vi "Teleop.vi"(10 "Match Info":T7={"Autonomous Elapsed Seconds"=0.0, "TeleOp Elapsed Seconds"=0.0, "Disabled Elapsed Seconds"=0.0, "Visited Autonomous"=FALSE, "Visited TeleOp"=FALSE, "Visited Disabled"=FALSE, "Autonomous Settings"={"Autonomous Style"=enum."Independent", "VI Refnum"=refnum}}, 11 "Call Context":T8) -> ()   [LabVIEW 2013]
doc: "This VI is called for each TeleOp packet received from the DS where the robot is not disabled. It is often used to read from the joysticks and update I/O or to update setpoints for timed control loops. It should complete and return within 20 milliseconds or it may miss DS packets."
uses:
  <vilib>/Rock Robotics/WPI/DriverStation/WPI_DriverStationDerivedRobotMode.ctl
  <vilib>/Rock Robotics/WPI/DriverStation/WPI_DriverStationMatch Info.ctl
  <vilib>/Rock Robotics/WPI/Solenoid/WPI_SolenoidValue.ctl
  <vilib>/Rock Robotics/WPI/Relay/WPI_RelayValue.ctl
  Robot Global Data.vi
  <vilib>/Rock Robotics/Network Tables/SD Read Number.vi
  <vilib>/Rock Robotics/WPI/Joystick/WPI_JoystickGetSetRefNum.vi
  <vilib>/Rock Robotics/WPI/RobotDrive/WPI_RobotDriveGetSetRefNum.vi
  <vilib>/Rock Robotics/WPI/Solenoid/WPI_SolenoidSetEnum.vi
  <vilib>/Rock Robotics/WPI/Compressor/WPI_CompressorGetSetRefNum.vi
  <vilib>/Rock Robotics/WPI/Solenoid/WPI_SolenoidGetEnum.vi
panel:
  out "LockControls 2":bool
  in  "Mechanism Piston Forward 2":bool
  out "ManualOverridePistonStates":T2
  in  "TimingForCopilot":T3
  out "MovingBackwards":bool
  out "LockControls":bool
  out "MovingBackwardsEncoderReset":bool
  out "Waveform Chart 4":dbl(graph)
  out "Waveform Chart 3":dbl(graph)
  in  "Grabber Timer":dbl
  in  "GrabberCurrentTarget":dbl
  in  "HasGrabberBeenReset":bool
  in  "ToughBoxEncoderTopPosition":dbl
  in  "Current Grabber Status":T4(ring)
  in  "Run Grabber PID 2":bool
  out "Reed Switch 2":bool
  out "Reed Switch 1":bool
  out "Top Limit Tripped":bool
  out "Micro Switch":bool
  out "Bottom Limit Tripped":bool
  out "Axis Value  6":dbl
  out "Axis Value 5":dbl
  out "Axis Value 4":dbl
  in  "Grabber Axis Value":T5(ring)
  in  "Current Shooter Status":T6(ring)
  out "Waveform Chart":dbl(graph)
  out "Mechanism Moving Up":bool
  out "Mechanism Moving Down":bool
  out "Time Since Button Pressed":dbl
  in  "Manual Override Activated":bool
  in  "Button 2 Pressed":bool
  in  "Firing Pin Forward":bool
  in  "Mechanism Piston Forward":bool
  in  "Tick Taken":bool
  out "Time at Gather":dbl
  out "Timer for firing mech":dbl
  in  "Mechanism Status":string
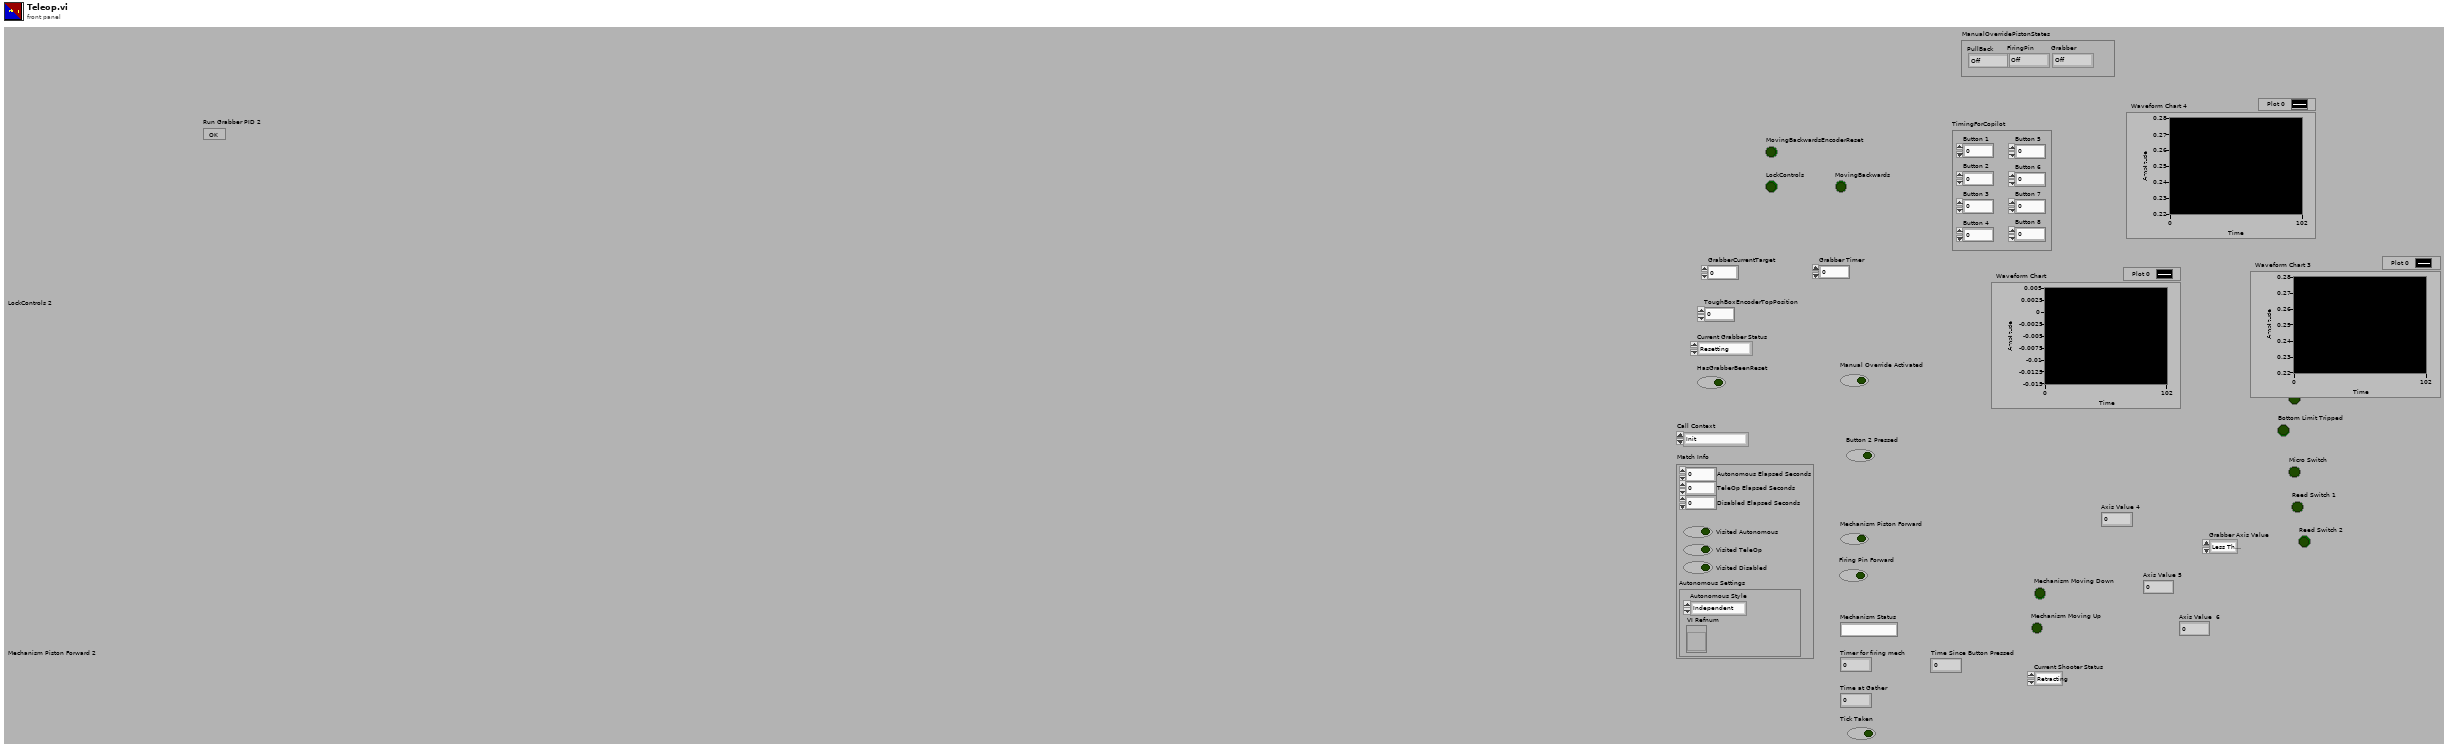
[diagram p1: front panel]
types:
  T1 = typedef "WPI_SolenoidValue.ctl" = enum16{"Off", "On", "Forward", "Reverse"}
  T2 = cluster{"PullBack":T1, "FiringPin":T1, "Grabber":T1}
  T3 = cluster{"Button 1":dbl, "Button 2":dbl, "Button 3":dbl, "Button 4":dbl, "Button 5":dbl, "Button 6":dbl, "Button 7":dbl, "Button 8":dbl}
  T4 = enum16{"Resetting", "Going Up", "Going Up Slow", "In Shooting Position", "Going Down", "Going Down Slow", "In Loading Position"}
  T5 = enum16{"Less Than Zero", "Greater Than Zero", "Equal To Zero"}
  T6 = enum16{"Retracting", "Firing", "Ready to fire", "Pulling back", "Just fired"}
  T7 = typedef "WPI_DriverStationMatch Info.ctl" = cluster{"Autonomous Elapsed Seconds":dbl, "TeleOp Elapsed Seconds":dbl, "Disabled Elapsed Seconds":dbl, "Visited Autonomous":bool, "Visited TeleOp":bool, "Visited Disabled":bool, "Autonomous Settings":cluster{"Autonomous Style":enum16{"Iterative", "Independent"}, "VI Refnum":refnum<vi>}}
  T8 = typedef "WPI_DriverStationDerivedRobotMode.ctl" = enum16{"Init", "Execute", "Stop"}
  T9 = enum16{"Resetting", "Going Up", "Going Up Slow", "In Shooting Position", "Going Down", "Going Down Slow", "In Loading Position", ""}
  T10 = typedef "WPI_JoystickDevRef.ctl" = cluster{"Device":T11}
  T11 = typedef "WPI_JoystickDeviceEnum.ctl" = enum16{"USB 1", "USB 2", "USB 3", "USB 4", "Kinect 1", "Kinect 2"}
  T12 = typedef "WPI_MotorControlDeviceRef.ctl" = cluster{"DeviceStatus":errorcluster, "Type":enum16{"PWM", "CAN"}, "PWM":cluster{"Digital Module":T13, "PWM Channel":T14, "DeadBand":T15}, "CAN":cluster{"Device Number":u8, "Control Mode":T16, "Semaphore":T17, "Max Vout":dbl}, "Invert":bool, "TransformRef":T18, "InvTransformRef":T18}
  T13 = typedef "FPGA_TypedefDigitalModule.ctl" = enum16{"Digital Module 1", "Digital Module 2"}
  T14 = typedef "FPGA_DIOPWMChannel.ctl" = enum8{"PWM 1", "PWM 2", "PWM 3", "PWM 4", "PWM 5", "PWM 6", "PWM 7", "PWM 8", "PWM 9", "PWM 10", "Invalid"}
  T15 = typedef "WPI_PWMDeadband.ctl" = cluster{"Name":string, "maxPositivePwm":i32, "minPositivePwm":i32, "centerPwm":i32, "maxNegativePwm":i32, "minNegativePwm":i32, "angularRange":u16}
  T16 = typedef "WPI_CANJaguar_ControlMode.ctl" = enum8{"Percent VBus", "Current", "Speed", "Position", "Voltage"}
  T17 = typedef "Semaphore RefNum" = refnum<k1>
  T18 = typedef "WPI_PWMTransform_ConPane.ctl" = refnum<vi>
  T19 = typedef "WPI_SolenoidDevRef.ctl" = cluster{"DevStatus":errorcluster, "Solenoid Module":T20, "Forward Solenoid Channel":T21, "Reverse Solenoid Channel":T21}
  T20 = typedef "FPGA_TypedefSolenoidModule.ctl" = enum16{"Solenoid Module 1", "Solenoid Module 2"}
  T21 = typedef "WPI_SolenoidChannel.ctl" = enum8{"Solenoid 1", "Solenoid 2", "Solenoid 3", "Solenoid 4", "Solenoid 5", "Solenoid 6", "Solenoid 7", "Solenoid 8", "Invalid"}
  T22 = typedef "WPI_JoystickButtonState.ctl" = cluster{"Button 1":bool, "Button 2":bool, "Button 3":bool, "Button 4":bool, "Button 5":bool, "Button 6":bool, "Button 7":bool, "Button 8":bool, "Button 9":bool, "Button 10":bool, "Button 11":bool, "Button 12":bool}
  T23 = typedef "WPI_DigitalInputDevRef.ctl" = cluster{"DevStatus":errorcluster, "DIO Channel":T24, "Digital Module":T13}
  T24 = typedef "FPGA_DIOChannel.ctl" = enum8{"DIO 1", "DIO 2", "DIO 3", "DIO 4", "DIO 5", "DIO 6", "DIO 7", "DIO 8", "DIO 9", "DIO 10", "DIO 11", "DIO 12", "DIO 13", "DIO 14", "Invalid"}
  T25 = typedef "WPI_EncoderDevRef.ctl" = cluster{"DevStatus":errorcluster, "EncoderIndex":T26, "CounterIndex":T27, "DistancePerCount":dbl, "Decoding Type":T28}
  T26 = typedef "FPGA_EncoderIdx.ctl" = enum8{"Enc 0", "Enc 1", "Enc 2", "Enc 3", "Invalid"}
  T27 = typedef "FPGA_CounterCtrSystemIndex.ctl" = enum8{"Ctr 0", "Ctr 1", "Ctr 2", "Ctr 3", "Ctr 4", "Ctr 5", "Ctr 6", "Ctr 7", "Invalid"}
  T28 = typedef "WPI_EncoderType.ctl" = enum16{"1x", "2x", "4x"}
  T29 = typedef "WPI_RelayDevRef.ctl" = cluster{"DevStatus":errorcluster, "Relay Channel":T30, "Digital Module":T13, "Relay Direction":T31}
  T30 = typedef "FPGA_DIORelayChannel.ctl" = enum8{"Relay 1", "Relay 2", "Relay 3", "Relay 4", "Relay 5", "Relay 6", "Relay 7", "Relay 8", "Invalid"}
  T31 = typedef "WPI_RelayDirection.ctl" = enum16{"Both directions", "Forward only", "Reverse only"}
  T32 = typedef "WPI_CompressorDevRef.ctl" = cluster{"DevStatus":errorcluster, "DigitalInputDevRef":T23, "RelayDevRef":T29}
  T33 = typedef "WPI_RelayValue.ctl" = enum16{"Off", "On", "Forward", "Reverse"}
  T34 = typedef "WPI_AnalogChannelDevRef.ctl" = cluster{"DevStatus":errorcluster, "Analog Module":T35, "Analog Channel":T36}
  T35 = typedef "FPGA_TypedefAnalogModule.ctl" = enum16{"Analog Module 1", "Analog Module 2"}
  T36 = typedef "FPGA_AIChannel.ctl" = enum8{"AI 1", "AI 2", "AI 3", "AI 4", "AI 5", "AI 6", "AI 7", "AI 8", "Invalid"}
  T37 = typedef "WPI_ServoDeviceRef.ctl" = cluster{"DeviceStatus":errorcluster, "Digital Module":T13, "PWM Channel":T14, "DeadBand":T15}
  T38 = cluster{"axis 1 (x)":dbl, "axis 2 (y)":dbl, "axis 3 (throttle)":dbl, "axis 4":dbl, "axis 5":dbl, "axis 6":dbl}
  T39 = typedef "WPI_RobotDriveDevRef.ctl" = cluster{"DevStatus":errorcluster, "Motors[]":T12[], "Square Inputs":bool, "Max Output":dbl, "Isochronous":bool}
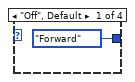
[diagram p3: hidden frame]
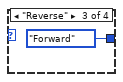
[diagram p4: hidden frame]
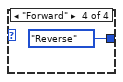
[diagram p5: hidden frame]
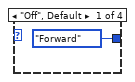
[diagram p7: hidden frame]
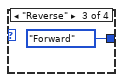
[diagram p8: hidden frame]
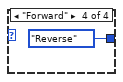
[diagram p9: hidden frame]
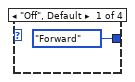
[diagram p11: hidden frame]
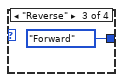
[diagram p12: hidden frame]
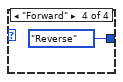
[diagram p13: hidden frame]
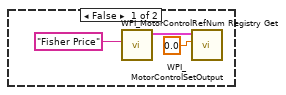
[diagram p15: hidden frame]
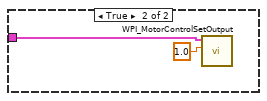
[diagram p16: hidden frame]
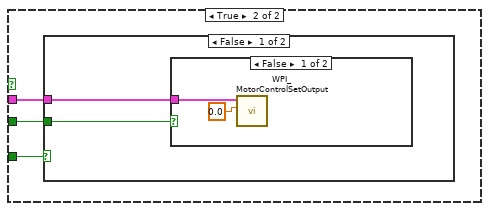
[diagram p17: hidden frame]
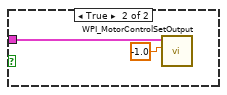
[diagram p18: hidden frame]
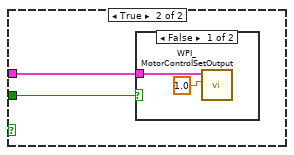
[diagram p19: hidden frame]
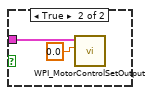
[diagram p20: hidden frame]
diagram:
  (unwired) FALSE
  (unwired) "This code sets the toggle rate used by the Periodic Tasks VI.  For teleop mode we flash the USER1 LED on the cRIO at a fast rate.  Look at the Periodic Tasks VI to see how this global value is used."
  (unwired) "This VI is called each time a TeleOp DS packet is received.  Use it to respond to new joystick or Driver Station values.\n\nCommon tasks include reading the joysticks and updating motors, and updating setpoints for periodic loops.\n\nYou can open I/O on the FIRST Call, or in the Begin.vi."
  # "Second joystick/copilot controls"
  # "Send information about the current state in the code to the drivers"
  # "one encoder"
  # "Top Limit Switch may need invert"
  # "one encoder"
  # "Check me!"
  # "Publish the Robot Drive Motor\nvalues to the dashboard"
  # "Each time we enter, report that\nwe are running teleop"
  # "Use to differentiate between\nFirst, Last, and Intermediate calls"
  # "Read Joystick X and Y values and update motor values"
  n1 = call <vilib>:"SD Read Boolean.vi"("Name"="Manual Mechanism Override") -> ("Boolean"=w100:bool)  [unwired: 8 in, 2 out]
  n2 = Not(x=w100) -> (.not. x?=w86:bool)
  n3 = local write "Firing Pin Forward"(FALSE) -> ()
  n4 = call <vilib>:"WPI_DriverStationReport Robot Code State.vi"("TeleOp"=TRUE ("Autonomous")) -> ()  [unwired: 10 in, 1 out]
  n5 = global write "Robot Global Data.vi" "LED toggle rate (ms)"(u32 100 ("LED ms toggle rate")) -> ()
  n6 = case shown="True" w86 {
    frame False {
    }
    frame True {
      n7 = local read "Current Grabber Status"() -> (w177:T4)
      n8 = case shown="\"Going Up Slow\"" w177 {
        frame "Going Up" {
          n9 = Divide(x=60.0 ("setpoint"), y=360.0) -> (x/y=w180:dbl)
          n10 = call "grabberpidinit.vi"("setpoint"=w180) -> ("Done? 2"=w181:bool)  [unwired: 10 in]
          n11 = case shown="True" w181 {
            tunnel: w180 -> [_ w182]
            frame False {
            }
            frame True {
              n12 = local write "GrabberCurrentTarget"(w182) -> ()
              n13 = local write "Current Grabber Status"(T4."Going Up Slow" ("Current Grabber Status")) -> ()
            }
          }
        }
        frame "In Loading Position" {
          # "Change to the UltraSonic Sensor\nwhen possible"
          n14 = call <vilib>:"WPI_JoystickRefNum Registry Get.vi"("refnum name"="Joystick 1") -> ("JoystickDevRef"=w186:T10)  [unwired: 1 in, 9 out]
          n15 = call <vilib>:"WPI_MotorControlRefNum Registry Get.vi"("refnum name"="Snowblower") -> ("MotorControlDevRef"=w193:T12)  [unwired: 9 in, 1 out]
          n16 = call <vilib>:"WPI_MotorControlSetOutput.vi"("Output"=1.0, "MotorControlDevRef"=w193) -> ()  [unwired: 7 in, 3 out]
          n17 = call <vilib>:"WPI_SolenoidRefNum Registry Get.vi"("refnum name"="Grabber Pistons Solenoid") -> ("error out"=w190:errorcluster, "SolenoidDevRef"=w189:T19)  [unwired: 9 in]
          n18 = call-poly <vilib>:"WPI_SolenoidSet.vi"("error in (no error)"=w190, "Value"=WPI_SolenoidValue."Reverse", "SolenoidDevRef"=w189) -> ()  [unwired: 7 in, 2 out]
          n19 = call <vilib>:"WPI_JoystickGet.vi"("JoystickDevRef"=w186) -> ("Buttons"=w185:T22)  [unwired: 1 in, 5 out]
          n20 = Unbundle By Name(w185) -> ("Button 4"=w184:bool)
          n21 = case shown="True" w184 {
            frame False {
            }
            frame True {
              n22 = local write "Current Grabber Status"(T4."Going Up" ("Current Grabber Status")) -> ()
            }
          }
        }
        frame "Going Down" {
          n23 = Divide(x=15.0, y=360.0) -> (x/y=w200:dbl)
          n24 = call "grabberpidinit.vi"("setpoint"=w200) -> ("Done? 2"=w201:bool)  [unwired: 10 in]
          n25 = case shown="True" w201 {
            tunnel: w200 -> [_ w206]
            frame False {
            }
            frame True {
              n26 = local write "GrabberCurrentTarget"(w206) -> ()
              n27 = local write "Current Grabber Status"(T4."Going Down Slow" ("Current Grabber Status")) -> ()
            }
          }
          n28 = call <vilib>:"WPI_DigitalInputRefNum Registry Get.vi"("refnum name"="Bottom Limit Switch") -> ("error out"=w198:errorcluster, "DigitalInputDevRef"=w197:T23)  [unwired: 9 in]
          n29 = call <vilib>:"WPI_DigitalInputGetValue.vi"("error in (no error)"=w198, "DigitalInputDevRef"=w197) -> ("Value"=w196:bool)  [unwired: 7 in, 2 out]
          n30 = case shown="True" w196 {
            frame False {
            }
            frame True {
              n31 = local write "Current Grabber Status"(T4."Going Down Slow" ("Current Grabber Status")) -> ()
            }
          }
        }
        frame "In Shooting Position" {
          n32 = call <vilib>:"WPI_JoystickRefNum Registry Get.vi"("refnum name"="Joystick 1") -> ("JoystickDevRef"=w209:T10)  [unwired: 1 in, 9 out]
          n33 = call <vilib>:"WPI_JoystickGet.vi"("JoystickDevRef"=w209) -> ("Buttons"=w208:T22)  [unwired: 1 in, 5 out]
          n34 = Unbundle By Name(w208) -> ("Button 1"=w207:bool)
          n35 = case shown="True" w207 {
            frame False {
            }
            frame True {
              n36 = local write "Current Grabber Status"(T9."Going Down" ("Current Grabber Status")) -> ()
            }
          }
        }
        frame "Going Down Slow" {
          n37 = call "grabberpidspeed.vi"("setpoint"=-20.0) -> ()  [unwired: 10 in, 1 out]
          n38 = call <vilib>:"WPI_DigitalInputRefNum Registry Get.vi"("refnum name"="Bottom Limit Switch") -> ("DigitalInputDevRef"=w214:T23)  [unwired: 9 in, 1 out]
          n39 = call <vilib>:"WPI_DigitalInputGetValue.vi"("DigitalInputDevRef"=w214) -> ("Value"=w213:bool)  [unwired: 8 in, 2 out]
          n40 = case shown="True" w213 {
            frame False {
            }
            frame True {
              n41 = local write "Current Grabber Status"(T4."In Loading Position" ("Current Grabber Status")) -> ()
            }
          }
        }
        frame "Going Up Slow" {
          n42 = call "grabberpidspeed.vi"("setpoint"=20.0) -> ()  [unwired: 10 in, 1 out]
          n43 = call <vilib>:"WPI_DigitalInputRefNum Registry Get.vi"("refnum name"="Top Limit Switch") -> ("DigitalInputDevRef"=w219:T23)  [unwired: 9 in, 1 out]
          n44 = call <vilib>:"WPI_DigitalInputGetValue.vi"("DigitalInputDevRef"=w219) -> ("Value"=w218:bool)  [unwired: 8 in, 2 out]
          n45 = case shown="True" w218 {
            frame False {
            }
            frame True {
              n46 = local write "Current Grabber Status"(T4."In Shooting Position" ("Current Grabber Status")) -> ()
            }
          }
        }
        frame "Resetting", Default {
          n47 = call "grabberpidspeed.vi"("setpoint"=-20.0) -> ()  [unwired: 10 in, 1 out]
          n48 = call <vilib>:"WPI_DigitalInputRefNum Registry Get.vi"("refnum name"="Bottom Limit Switch") -> ("DigitalInputDevRef"=w226:T23)  [unwired: 9 in, 1 out]
          n49 = call <vilib>:"WPI_DigitalInputGetValue.vi"("DigitalInputDevRef"=w226) -> ("Value"=w224:bool)  [unwired: 8 in, 2 out]
          n50 = Not(x=w224) -> (.not. x?=w223:bool)
          n51 = case shown="True" w223 {
            frame False {
            }
            frame True {
              n52 = local write "Current Grabber Status"(T9."In Loading Position" ("Current Grabber Status")) -> ()
              n53 = call <vilib>:"WPI_EncoderRefNum Registry Get.vi"("refnum name"="Tough Box Encoder") -> ("error out"=w229:errorcluster, "EncoderDevRef"=w228:T25)  [unwired: 9 in]
              n54 = call <vilib>:"WPI_EncoderReset.vi"("error in (no error)"=w229, "EncoderDevRef"=w228) -> ()  [unwired: 8 in, 2 out]
            }
          }
          n55 = Tick Count (ms)() -> ()  [unwired: 1 out]
        }
      }
    }
  }
  n56 = Unbundle By Name("Match Info") -> ()  [unwired: 1 out]
  n57 = call <vilib>:"SD Read Boolean.vi"("Name"="Light Ring On") -> ("Boolean"=w106:bool)  [unwired: 8 in, 2 out]
  n58 = call <vilib>:"WPI_RelayRefNum Registry Get.vi"("refnum name"="Light Ring") -> ("RelayDevRef"=w105:T29)  [unwired: 9 in, 1 out]
  n59 = call <vilib>:"WPI_DigitalInputRefNum Registry Get.vi"("refnum name"="Reed Switch 1") -> ("DigitalInputDevRef"=w124:T23)  [unwired: 9 in, 1 out]
  n60 = call <vilib>:"WPI_DigitalInputRefNum Registry Get.vi"("refnum name"="Reed Switch 2") -> ("DigitalInputDevRef"=w117:T23)  [unwired: 9 in, 1 out]
  n61 = call <vilib>:"WPI_DigitalInputRefNum Registry Get.vi"("refnum name"="Reed Switch 2") -> ("DigitalInputDevRef"=w121:T23)  [unwired: 9 in, 1 out]
  n62 = call <vilib>:"WPI_DigitalInputRefNum Registry Get.vi"("refnum name"="Micro Switch 1") -> ("DigitalInputDevRef"=w134:T23)  [unwired: 9 in, 1 out]
  n63 = call <vilib>:"WPI_DigitalInputRefNum Registry Get.vi"("refnum name"="Micro Switch 1") -> ("DigitalInputDevRef"=w113:T23)  [unwired: 9 in, 1 out]
  n64 = call <vilib>:"WPI_DigitalInputRefNum Registry Get.vi"("refnum name"="Top Limit Switch") -> ("DigitalInputDevRef"=w127:T23)  [unwired: 9 in, 1 out]
  n65 = call <vilib>:"SD Read Boolean.vi"("Name"="Compressor On/Off") -> ("Boolean"=w136:bool)  [unwired: 8 in, 2 out]
  n66 = call <vilib>:"WPI_CompressorRefNum Registry Get.vi"("refnum name"="Compressor") -> ("CompressorDevRef"=w137:T32)  [unwired: 9 in, 1 out]
  n67 = call <vilib>:"WPI_DigitalInputRefNum Registry Get.vi"("refnum name"="Bottom Limit Switch") -> ("DigitalInputDevRef"=w142:T23)  [unwired: 9 in, 1 out]
  n68 = case shown="False" w106 {
    tunnel: w105 -> [w231 w234]
    frame False {
      n69 = call <vilib>:"WPI_RelaySet.vi"("RelayValue"=WPI_RelayValue."Off", "RelayDevRef"=w231) -> ()  [unwired: 8 in, 2 out]
    }
    frame True {
      n70 = call <vilib>:"WPI_RelaySet.vi"("RelayValue"=WPI_RelayValue."Forward", "RelayDevRef"=w234) -> ()  [unwired: 8 in, 2 out]
    }
  }
  n71 = call <vilib>:"WPI_DigitalInputGetValue.vi"("DigitalInputDevRef"=w124) -> ("Value"=→"Reed Switch 1":bool)  [unwired: 8 in, 2 out]
  n72 = call <vilib>:"WPI_DigitalInputGetValue.vi"("DigitalInputDevRef"=w117) -> ("Value"=w116:bool)  [unwired: 8 in, 2 out]
  n73 = call <vilib>:"WPI_DigitalInputGetValue.vi"("DigitalInputDevRef"=w121) -> ("Value"=→"Reed Switch 2":bool)  [unwired: 8 in, 2 out]
  n74 = call <vilib>:"WPI_DigitalInputGetValue.vi"("DigitalInputDevRef"=w134) -> ("Value"=→"Micro Switch":bool)  [unwired: 8 in, 2 out]
  n75 = call <vilib>:"WPI_DigitalInputGetValue.vi"("DigitalInputDevRef"=w113) -> ("Value"=w112:bool)  [unwired: 8 in, 2 out]
  n76 = call <vilib>:"WPI_DigitalInputGetValue.vi"("DigitalInputDevRef"=w127) -> ("Value"=→"Top Limit Tripped":bool)  [unwired: 8 in, 2 out]
  n77 = call <vilib>:"WPI_AnalogChannelRefNum Registry Get.vi"("refnum name"="Grabber Ultrasonic Sensor") -> ("AIDeviceRef"=w103:T34)  [unwired: 9 in, 1 out]
  n78 = case shown="False" w136 {
    tunnel: w137 -> [w235 w236]
    frame False {
      n79 = call <vilib>:"WPI_CompressorStop.vi"("CompressorDevRef"=w235) -> ()  [unwired: 9 in, 2 out]
    }
    frame True {
      n80 = call <vilib>:"WPI_CompressorStart.vi"("CompressorDevRef"=w236) -> ()  [unwired: 9 in, 2 out]
    }
  }
  n81 = call <vilib>:"WPI_DigitalInputGetValue.vi"("DigitalInputDevRef"=w142) -> ("Value"=→"Bottom Limit Tripped":bool)  [unwired: 8 in, 2 out]
  n82 = Not(x=w116) -> (.not. x?=w115:bool)
  n83 = call-poly <vilib>:"SD Read Value.vi"("Name"="Camera Pitch Control") -> ("Numeric"=w151:dbl)  [unwired: 8 in, 2 out]
  n84 = Not(x=w112) -> (.not. x?=w111:bool)
  n85 = call <vilib>:"WPI_ServoRefNum Registry Get.vi"("refnum name"="Camera Pitch Servo") -> ("ServoDeviceRef"=w152:T37)  [unwired: 9 in, 1 out]
  n86 = call-poly <vilib>:"SD Read Value.vi"("Name"="Camera Rotation Control") -> ("Numeric"=w155:dbl)  [unwired: 8 in, 2 out]
  n87 = call <vilib>:"WPI_AnalogChannelGetVoltage.vi"("AIDeviceRef"=w103) -> ("Voltage"=→"Waveform Chart":dbl)  [unwired: 8 in, 2 out]
  n88 = call <vilib>:"WPI_ServoRefNum Registry Get.vi"("refnum name"="Camera Rotation Servo") -> ("ServoDeviceRef"=w154:T37)  [unwired: 9 in, 1 out]
  n89 = call <vilib>:"SD Write Boolean.vi"("Boolean"=w115, "Name"="Are Drawback Pistons Extended") -> ()  [unwired: 8 in, 2 out]
  n90 = call <vilib>:"SD Write Boolean.vi"("Boolean"=w111, "Name"="Is The Firing Pin Piston Extended") -> ()  [unwired: 8 in, 2 out]
  n91 = call <vilib>:"SD Read Boolean.vi"("Name"="Manual Mechanism Override") -> ("Boolean"=w145:bool)  [unwired: 8 in, 2 out]
  n92 = call <vilib>:"WPI_JoystickRefNum Registry Get.vi"("refnum name"="Joystick 1") -> ("JoystickDevRef"=w164:T10)  [unwired: 1 in, 9 out]
  n93 = call <vilib>:"WPI_ServoSetAngle.vi"("Angle"=w151, "ServoDeviceRef"=w152) -> ()  [unwired: 8 in, 2 out]
  n94 = call <vilib>:"WPI_ServoSetAngle.vi"("Angle"=w155, "ServoDeviceRef"=w154) -> ()  [unwired: 8 in, 2 out]
  n95 = call <vilib>:"SD Read Boolean.vi"("Name"="Drawback Pistons Activated") -> ("Boolean"=w131:bool)  [unwired: 8 in, 2 out]
  n96 = Not(x=w145) -> (.not. x?=w130:bool)
  n97 = call <vilib>:"WPI_JoystickGet.vi"("JoystickDevRef"=w164) -> ("Buttons"=w163:T22, "Axes"=w161:T38)  [unwired: 1 in, 4 out]
  n98 = call <vilib>:"WPI_JoystickRefNum Registry Get.vi"("refnum name"="Joystick 1") -> ("JoystickDevRef"=w80:T10)  [unwired: 1 in, 9 out]
  n99 = Unbundle By Name(w163) -> ("Button 3"=w93:bool, "Button 5"=w109:bool, "Button 6"=w110:bool)  [unwired: 2 out]
  n100 = And(x=w130, y=w131) -> (x .and. y?=w129:bool)
  n101 = Unbundle By Name(w161) -> ("axis 4"=→"Axis Value 4":dbl, "axis 5"=→"Axis Value 5":dbl, "axis 6"=→"Axis Value  6":dbl)
  n102 = call <vilib>:"WPI_MotorControlRefNum Registry Get.vi"("refnum name"="Snowblower") -> ("MotorControlDevRef"=w91:T12)  [unwired: 9 in, 1 out]
  n103 = local read "MovingBackwards"() -> (w75:bool)
  n104 = call <vilib>:"WPI_JoystickGet.vi"("JoystickDevRef"=w80) -> ("Buttons"=w79:T22)  [unwired: 1 in, 5 out]
  n105 = call <vilib>:"SD Read Boolean.vi"("Name"="Manual Mechanism Override") -> ("Boolean"=w73:bool)  [unwired: 8 in, 2 out]
  n106 = Unbundle By Name(w79) -> ("Button 3"=w76:bool)
  n107 = case shown="False" w73 {
    tunnel: w110 -> [_ w245]
    tunnel: w109 -> [w237 w244]
    tunnel: w91 -> [w238 w243]
    frame False {
      n108 = case shown="False" w237 {
        tunnel: w238 -> [w239 w241]
        frame False {
          n109 = call <vilib>:"WPI_MotorControlSetOutput.vi"("Output"=-1.0, "MotorControlDevRef"=w239) -> ()  [unwired: 7 in, 3 out]
        }
        frame True {
          n110 = call <vilib>:"WPI_MotorControlSetOutput.vi"("Output"=1.0, "MotorControlDevRef"=w241) -> ()  [unwired: 7 in, 3 out]
        }
      }
    }
    frame True {
      n111 = case shown="False" w245 {
        tunnel: w244 -> [w247 w253]
        tunnel: w243 -> [w246 w252]
        frame False {
          n112 = case shown="False" w247 {
            tunnel: w246 -> [w249 w251]
            frame False {
              n113 = call <vilib>:"WPI_MotorControlSetOutput.vi"("Output"=0.0, "MotorControlDevRef"=w249) -> ()  [unwired: 7 in, 3 out]
            }
            frame True {
              n114 = call <vilib>:"WPI_MotorControlSetOutput.vi"("Output"=-1.0, "MotorControlDevRef"=w251) -> ()  [unwired: 7 in, 3 out]
            }
          }
        }
        frame True {
          n115 = case shown="False" w253 {
            tunnel: w252 -> [w255 w257]
            frame False {
              n116 = call <vilib>:"WPI_MotorControlSetOutput.vi"("Output"=1.0, "MotorControlDevRef"=w255) -> ()  [unwired: 7 in, 3 out]
            }
            frame True {
              n117 = call <vilib>:"WPI_MotorControlSetOutput.vi"("Output"=0.0, "MotorControlDevRef"=w257) -> ()  [unwired: 7 in, 3 out]
            }
          }
        }
      }
    }
  }
  n118 = case shown="True" w75 {
    frame False {
      n119 = local write "LockControls"(FALSE) -> ()
    }
    frame True {
      n120 = local read "MovingBackwardsEncoderReset"() -> (w287:bool)
      n121 = local write "LockControls"(TRUE) -> ()
      n122 = call <vilib>:"WPI_EncoderRefNum Registry Get.vi"("refnum name"="Left Drive Encoder") -> ("error out"=w272:errorcluster, "EncoderDevRef"=w263:T25)  [unwired: 9 in]
      n123 = call <vilib>:"WPI_EncoderGet.vi"("error in (no error)"=w272, "EncoderDevRef"=w263) -> ("Distance"=w264:dbl)  [unwired: 4 in, 5 out]
      n124 = call <vilib>:"WPI_EncoderRefNum Registry Get.vi"("refnum name"="Right Drive Encoder") -> ("error out"=w273:errorcluster, "EncoderDevRef"=w274:T25)  [unwired: 9 in]
      n125 = call <vilib>:"WPI_EncoderGet.vi"("error in (no error)"=w273, "EncoderDevRef"=w274) -> ("Distance"=w276:dbl)  [unwired: 4 in, 5 out]
      n126 = Add(x=w264, y=w276) -> (x+y=w277:dbl)
      n127 = case shown="False" w287 {
        frame False {
          n128 = call <vilib>:"WPI_EncoderRefNum Registry Get.vi"("refnum name"="Left Drive Encoder") -> ("error out"=w300:errorcluster, "EncoderDevRef"=w299:T25)  [unwired: 9 in]
          n129 = call <vilib>:"WPI_EncoderRefNum Registry Get.vi"("refnum name"="Right Drive Encoder") -> ("error out"=w303:errorcluster, "EncoderDevRef"=w302:T25)  [unwired: 9 in]
          n130 = local write "MovingBackwardsEncoderReset"(TRUE ("MovingBackwardsEncoderReset")) -> ()
          n131 = call <vilib>:"WPI_EncoderReset.vi"("error in (no error)"=w300, "EncoderDevRef"=w299) -> ()  [unwired: 8 in, 2 out]
          n132 = call <vilib>:"WPI_EncoderReset.vi"("error in (no error)"=w303, "EncoderDevRef"=w302) -> ()  [unwired: 8 in, 2 out]
        }
        frame True {
        }
      }
      n133 = Divide(x=w277, y=2.0) -> (x/y=w281:dbl)
      n134 = call "distancepidinit.vi"("Distance From Target"=-8.0) -> ("Done?"=w259:bool)  [unwired: 10 in]
      n135 = case shown="True" w259 {
        frame False {
        }
        frame True {
          n136 = local write "MovingBackwardsEncoderReset"(FALSE ("MovingBackwardsEncoderReset")) -> ()
          n137 = local write "MovingBackwards"(FALSE ("MovingBackwards")) -> ()
        }
      }
      n138 = Multiply(x=6.0, y=3.141592653589793) -> (x*y=w284:dbl)
      n139 = Divide(x=w281, y=360.0) -> (x/y=w283:dbl)
      n140 = Multiply(x=w283, y=w284) -> (x*y=w285:dbl)
      n141 = Divide(x=w285, y=12.0) -> (x/y=w271:dbl)
      n142 = Multiply(x=w271, y=0.48) -> (x*y=w265:dbl)
      n143 = Greater?(x=w265, y=-5.0) -> (0:w266:bool)
      n144 = Greater?(x=w265, y=-4.0) -> (0:w268:bool)
      n145 = case shown="True" w266 {
        frame False {
        }
        frame True {
          n146 = call <vilib>:"WPI_SolenoidRefNum Registry Get.vi"("refnum name"="Firing Pin") -> ("error out"=w290:errorcluster, "SolenoidDevRef"=w291:T19)  [unwired: 9 in]
          n147 = call-poly <vilib>:"WPI_SolenoidSet.vi"("error in (no error)"=w290, "Value"=WPI_SolenoidValue."Reverse", "SolenoidDevRef"=w291) -> ()  [unwired: 7 in, 2 out]
        }
      }
      n148 = case shown="True" w268 {
        frame False {
        }
        frame True {
          n149 = call <vilib>:"WPI_SolenoidRefNum Registry Get.vi"("refnum name"="Grabber Pistons") -> ("error out"=w294:errorcluster, "SolenoidDevRef"=w295:T19)  [unwired: 9 in]
          n150 = call-poly <vilib>:"WPI_SolenoidSet.vi"("error in (no error)"=w294, "Value"=WPI_SolenoidValue."Forward", "SolenoidDevRef"=w295) -> ()  [unwired: 7 in, 2 out]
        }
      }
    }
  }
  n151 = case shown="True" w76 {
    frame False {
    }
    frame True {
      n152 = local write "MovingBackwards"(TRUE ("MovingBackwards")) -> ()
    }
  }
  n153 = local read "Current Grabber Status"() -> (w96:T4)
  n154 = local read "Current Shooter Status"() -> (w97:T6)
  n155 = case shown="True" w129 {
    tunnel: w93 -> [_ w306]
    frame False {
    }
    frame True {
      n156 = case shown="\"Pulling back\"" "Current Shooter Status" {
        tunnel: w306 -> [_ w314 _ _ _]
        frame "Firing" {
          n157 = Tick Count (ms)() -> (millisecond timer value=w308:u32)
          n158 = local write "Current Shooter Status"(T6."Just fired" ("Current Shooter Status")) -> ()
          n159 = call <vilib>:"WPI_SolenoidRefNum Registry Get.vi"("refnum name"="Firing Pin Solenoid") -> ("error out"=w312:errorcluster, "SolenoidDevRef"=w311:T19)  [unwired: 9 in]
          n160 = call-poly <vilib>:"WPI_SolenoidSet.vi"("error in (no error)"=w312, "Value"=WPI_SolenoidValue."Reverse", "SolenoidDevRef"=w311) -> ()  [unwired: 7 in, 2 out]
          n161 = local write "Timer for firing mech"(w308) -> ()
        }
        frame "Ready to fire" {
          # "Button one is pressed, so fire"
          n162 = case shown="True" w314 {
            frame False {
            }
            frame True {
              n163 = local write "Current Shooter Status"(T6."Firing" ("Current Shooter Status")) -> ()
            }
          }
        }
        frame "Pulling back" {
          # "Need to invert reed switch 2"
          n164 = call <vilib>:"WPI_DigitalInputRefNum Registry Get.vi"("refnum name"="Reed Switch 2") -> ("error out"=w317:errorcluster, "DigitalInputDevRef"=w318:T23)  [unwired: 9 in]
          n165 = call <vilib>:"WPI_DigitalInputGetValue.vi"("error in (no error)"=w317, "DigitalInputDevRef"=w318) -> ("Value"=w316:bool)  [unwired: 7 in, 2 out]
          n166 = call <vilib>:"WPI_SolenoidRefNum Registry Get.vi"("refnum name"="Drawback Pistons") -> ("error out"=w322:errorcluster, "SolenoidDevRef"=w321:T19)  [unwired: 9 in]
          n167 = call <vilib>:"WPI_SolenoidRefNum Registry Get.vi"("refnum name"="Firing Pin Solenoid") -> ("error out"=w326:errorcluster, "SolenoidDevRef"=w325:T19)  [unwired: 9 in]
          n168 = call-poly <vilib>:"WPI_SolenoidSet.vi"("error in (no error)"=w322, "Value"=WPI_SolenoidValue."Forward", "SolenoidDevRef"=w321) -> ()  [unwired: 7 in, 2 out]
          n169 = case shown="True" w316 {
            frame False {
            }
            frame True {
              n170 = Tick Count (ms)() -> (millisecond timer value=w328:u32)
              n171 = local write "Timer for firing mech"(w328) -> ()
              n172 = local write "Current Shooter Status"(T6."Retracting" ("Current Shooter Status")) -> ()
            }
          }
          n173 = call-poly <vilib>:"WPI_SolenoidSet.vi"("error in (no error)"=w326, "Value"=WPI_SolenoidValue."Reverse", "SolenoidDevRef"=w325) -> ()  [unwired: 7 in, 2 out]
        }
        frame "Retracting" {
          n174 = local read "Timer for firing mech"() -> (w343:dbl)
          n175 = call <vilib>:"WPI_DigitalInputRefNum Registry Get.vi"("refnum name"="Reed Switch 1") -> ("error out"=w337:errorcluster, "DigitalInputDevRef"=w338:T23)  [unwired: 9 in]
          n176 = call <vilib>:"WPI_DigitalInputGetValue.vi"("error in (no error)"=w337, "DigitalInputDevRef"=w338) -> ("Value"=w330:bool)  [unwired: 7 in, 2 out]
          n177 = call <vilib>:"WPI_SolenoidRefNum Registry Get.vi"("refnum name"="Firing Pin Solenoid") -> ("error out"=w346:errorcluster, "SolenoidDevRef"=w345:T19)  [unwired: 9 in]
          n178 = Not(x=w330) -> (.not. x?=w331:bool)
          n179 = call-poly <vilib>:"WPI_SolenoidSet.vi"("error in (no error)"=w346, "Value"=WPI_SolenoidValue."Forward", "SolenoidDevRef"=w345) -> ()  [unwired: 7 in, 2 out]
          n180 = Tick Count (ms)() -> (millisecond timer value=w342:u32)
          n181 = case shown="True" w331 {
            frame False {
            }
            frame True {
              n182 = local write "Current Shooter Status"(T6."Ready to fire" ("Current Shooter Status")) -> ()
            }
          }
          n183 = Subtract(x=w342, y=w343) -> (x-y=w333:dbl)
          n184 = Greater Or Equal?(x=w333, y=1000) -> (x >= y?=w335:bool)
          n185 = call <vilib>:"WPI_SolenoidRefNum Registry Get.vi"("refnum name"="Drawback Pistons") -> ("SolenoidDevRef"=w340:T19)  [unwired: 9 in, 1 out]
          n186 = And(x=TRUE, y=w335) -> (x .and. y?=w336:bool)
          n187 = case shown="False" w336 {
            tunnel: w340 -> [w349 w351]
            frame False {
              n188 = call-poly <vilib>:"WPI_SolenoidSet.vi"("Value"=WPI_SolenoidValue."Forward", "SolenoidDevRef"=w349) -> ()  [unwired: 8 in, 2 out]
            }
            frame True {
              n189 = call-poly <vilib>:"WPI_SolenoidSet.vi"("Value"=WPI_SolenoidValue."Reverse", "SolenoidDevRef"=w351) -> ()  [unwired: 8 in, 2 out]
            }
          }
        }
        frame "Just fired", Default {
          # "When MicroSwitch is \nadded, Change this \nto read from that"
          n190 = local read "Timer for firing mech"() -> (w363:dbl)
          n191 = call <vilib>:"WPI_SolenoidRefNum Registry Get.vi"("refnum name"="Firing Pin Solenoid") -> ("error out"=w360:errorcluster, "SolenoidDevRef"=w359:T19)  [unwired: 9 in]
          n192 = Tick Count (ms)() -> (millisecond timer value=w362:u32)
          n193 = call-poly <vilib>:"WPI_SolenoidSet.vi"("error in (no error)"=w360, "Value"=WPI_SolenoidValue."Reverse", "SolenoidDevRef"=w359) -> ()  [unwired: 7 in, 2 out]
          n194 = Subtract(x=w362, y=w363) -> (x-y=w354:dbl)
          n195 = Greater Or Equal?(x=w354, y=3000) -> (x >= y?=w357:bool)
          n196 = And(x=TRUE, y=w357) -> (x .and. y?=w356:bool)
          n197 = case shown="True" w356 {
            frame False {
            }
            frame True {
              n198 = local write "Current Shooter Status"(T6."Pulling back" ("Current Shooter Status")) -> ()
            }
          }
        }
      }
    }
  }
  n199 = case shown="\"Resetting\", Default" w96 {
    tunnel: ["Resetting" "Going Up" "Going Up Slow" "In Shooting Position" "Going Down" "Going Down Slow" "In Loading Position"] -> w95
    frame "Resetting", Default {
    }
    frame "Going Up" {
    }
    frame "Going Up Slow" {
    }
    frame "In Shooting Position" {
    }
    frame "Going Down" {
    }
    frame "Going Down Slow" {
    }
    frame "In Loading Position" {
    }
  }
  n200 = case shown="\"Retracting\", Default" w97 {
    tunnel: ["Retracting" "Firing" "Ready to fire" "Pulling back" "Just fired"] -> w94
    frame "Retracting", Default {
    }
    frame "Firing" {
    }
    frame "Ready to fire" {
    }
    frame "Pulling back" {
    }
    frame "Just fired" {
    }
  }
  n201 = call <vilib>:"SD Write String.vi"("String"=w94, "Name"="Current Shooter Status") -> ()  [unwired: 8 in, 2 out]
  n202 = call <vilib>:"SD Write String.vi"("String"=w95, "Name"="Current Grabber Status") -> ()  [unwired: 8 in, 2 out]
  n203 = call <vilib>:"WPI_EncoderRefNum Registry Get.vi"("refnum name"="Right Drive Encoder") -> ("error out"=w90:errorcluster, "EncoderDevRef"=w89:T25)  [unwired: 9 in]
  n204 = call <vilib>:"WPI_EncoderGet.vi"("error in (no error)"=w90, "EncoderDevRef"=w89) -> ("Distance"=→"Waveform Chart 4":dbl)  [unwired: 4 in, 5 out]
  n205 = call <vilib>:"WPI_JoystickRefNum Registry Get.vi"("refnum name"="Joystick 2") -> ("JoystickDevRef"=w71:T10)  [unwired: 1 in, 9 out]
  n206 = call <vilib>:"WPI_JoystickGet.vi"("JoystickDevRef"=w71) -> ("Buttons"=w70:T22, "Axes"=w51:T38)  [unwired: 1 in, 4 out]
  n207 = Unbundle By Name(w51) -> ("axis 3 (throttle)"=w44:dbl, "axis 5"=w50:dbl)
  n208 = Negate(x=w50) -> (-x=w49:dbl)
  n209 = Multiply(x=w49, y=0.75) -> (x*y=w47:dbl)
  n210 = call <vilib>:"WPI_DigitalInputRefNum Registry Get.vi"("refnum name"="Micro Switch 1") -> ("DigitalInputDevRef"=w63:T23)  [unwired: 9 in, 1 out]
  n211 = Unbundle By Name(w70) -> ("Button 1"=w29:bool, "Button 2"=w11:bool, "Button 3"=w2:bool)  [unwired: 1 out]
  n212 = call <vilib>:"WPI_DigitalInputRefNum Registry Get.vi"("refnum name"="Bottom Limit Switch") -> ("DigitalInputDevRef"=w67:T23)  [unwired: 9 in, 1 out]
  n213 = call <vilib>:"WPI_DigitalInputGetValue.vi"("DigitalInputDevRef"=w63) -> ("Value"=w64:bool)  [unwired: 8 in, 2 out]
  n214 = call <vilib>:"WPI_DigitalInputRefNum Registry Get.vi"("refnum name"="Top Limit Switch") -> ("DigitalInputDevRef"=w60:T23)  [unwired: 9 in, 1 out]
  n215 = call <vilib>:"WPI_DigitalInputGetValue.vi"("DigitalInputDevRef"=w67) -> ("Value"=w55:bool)  [unwired: 8 in, 2 out]
  n216 = call <vilib>:"WPI_DigitalInputGetValue.vi"("DigitalInputDevRef"=w60) -> ("Value"=w52:bool)  [unwired: 8 in, 2 out]
  n217 = Not(x=w64) -> (.not. x?=w54:bool)
  n218 = Multiply(x=w44, y=0.4) -> (x*y=w45:dbl)
  n219 = local read "TimingForCopilot"() -> (w28:T3)
  n220 = Add(x=w47, y=w45) -> (x+y=w46:dbl)
  n221 = And(x=w55, y=w54) -> (x .and. y?=w53:bool)
  n222 = And(x=w52, y=w54) -> (x .and. y?=w58:bool)
  n223 = call <vilib>:"WPI_EncoderRefNum Registry Get.vi"("refnum name"="Tough Box Encoder") -> ("error out"=w85:errorcluster, "EncoderDevRef"=w84:T25)  [unwired: 9 in]
  n224 = Greater?(x=w46, y=0.01) -> (0:w59:bool)
  n225 = Less?(x=w46, y=-0.01) -> (x < y?=w66:bool)
  n226 = call <vilib>:"WPI_EncoderGet.vi"("error in (no error)"=w85, "EncoderDevRef"=w84) -> ("Distance"=→"Waveform Chart 3":dbl)  [unwired: 4 in, 5 out]
  n227 = And(x=w59, y=w58) -> (x .and. y?=w57:bool)
  n228 = Unbundle By Name(w28) -> ("Button 1"=w27:dbl, "Button 2"=w10:dbl, "Button 3"=w3:dbl)
  n229 = call <vilib>:"SD Read Boolean.vi"("Name"="Manual Mechanism Override") -> ("Boolean"=w36:bool)  [unwired: 8 in, 2 out]
  n230 = And(x=w53, y=w66) -> (x .and. y?=w56:bool)
  n231 = local read "LockControls"() -> (w78:bool)
  n232 = local read "ManualOverridePistonStates"() -> (w1:T2)
  n233 = Or(x=w56, y=w57) -> (x .or. y?=w41:bool)
  n234 = Tick Count (ms)() -> (millisecond timer value=w34:u32)
  n235 = Tick Count (ms)() -> (millisecond timer value=w21:u32)
  n236 = Tick Count (ms)() -> (millisecond timer value=w16:u32)
  n237 = call <vilib>:"SD Read Boolean.vi"("Name"="Grabber Limits Disabled") -> ("Boolean"=w39:bool)  [unwired: 8 in, 2 out]
  n238 = local read "Manual Override Activated"() -> (w37:bool)
  n239 = Or(x=w41, y=w39) -> (x .or. y?=w42:bool)
  n240 = Subtract(x=w34, y=w27) -> (x-y=w33:dbl)
  n241 = Subtract(x=w21, y=w10) -> (x-y=w20:dbl)
  n242 = Subtract(x=w16, y=w3) -> (x-y=w15:dbl)
  n243 = Not(x=w78) -> (.not. x?=w77:bool)
  n244 = Not Equal?(x=w37, y=w36) -> (x != y?=w35:bool)
  n245 = Greater?(x=w33, y=400.0) -> (0:w30:bool)
  n246 = Greater?(x=w20, y=400.0) -> (0:w17:bool)
  n247 = Greater?(x=w15, y=400.0) -> (0:w12:bool)
  n248 = Unbundle By Name(w1) -> ("PullBack"=w23:T1, "FiringPin"=w8:T1, "Grabber"=w4:T1)
  n249 = And(x=w30, y=w29) -> (x .and. y?=w31:bool)
  n250 = And(x=w17, y=w11) -> (x .and. y?=w18:bool)
  n251 = And(x=w12, y=w2) -> (x .and. y?=w13:bool)
  n252 = flat-sequence {
    tunnel: w35 -> [w377]
    frame #0 {
      n253 = case shown="True" w377 {
        frame False {
        }
        frame True {
          n254 = call <vilib>:"WPI_SolenoidRefNum Registry Get.vi"("refnum name"="Firing Pin") -> ("error out"=w384:errorcluster, "SolenoidDevRef"=w383:T19)  [unwired: 9 in]
          n255 = local read "ManualOverridePistonStates"() -> (w391:T2)
          n256 = call-poly <vilib>:"WPI_SolenoidGet.vi"("error in (no error)"=w384, "SolenoidDevRef"=w383) -> ("Value"=w382:T1)  [unwired: 7 in, 2 out]
          n257 = call <vilib>:"WPI_SolenoidRefNum Registry Get.vi"("refnum name"="Drawback Pistons") -> ("error out"=w388:errorcluster, "SolenoidDevRef"=w387:T19)  [unwired: 9 in]
          n258 = call <vilib>:"WPI_SolenoidRefNum Registry Get.vi"("refnum name"="Grabber Pistons") -> ("error out"=w380:errorcluster, "SolenoidDevRef"=w379:T19)  [unwired: 9 in]
          n259 = call-poly <vilib>:"WPI_SolenoidGet.vi"("error in (no error)"=w388, "SolenoidDevRef"=w387) -> ("Value"=w386:T1)  [unwired: 7 in, 2 out]
          n260 = call-poly <vilib>:"WPI_SolenoidGet.vi"("error in (no error)"=w380, "SolenoidDevRef"=w379) -> ("Value"=w378:T1)  [unwired: 7 in, 2 out]
          n261 = Bundle By Name(cluster=w391, "PullBack"=w386, "FiringPin"=w382, "Grabber"=w378) -> (w390:T2)
          n262 = local write "ManualOverridePistonStates"(w390) -> ()
        }
      }
    }
  }
  n263 = case shown="True" w31 {
    tunnel: w27 -> [w393 _]
    tunnel: [w393 w396] -> w26
    tunnel: w23 -> [w392 w395]
    tunnel: [w392 w394] -> w22
    frame False {
    }
    frame True {
      n264 = case shown="\"On\"" w395 {
        tunnel: [WPI_SolenoidValue."Forward" ("FiringPin") WPI_SolenoidValue."Reverse" ("FiringPin") WPI_SolenoidValue."Forward" ("FiringPin") WPI_SolenoidValue."Reverse" ("FiringPin")] -> w394
        frame "Off", Default {
        }
        frame "On" {
        }
        frame "Reverse" {
        }
        frame "Forward" {
        }
      }
      n265 = Tick Count (ms)() -> (millisecond timer value=w396:u32)
    }
  }
  n266 = case shown="True" w18 {
    tunnel: w10 -> [w402 _]
    tunnel: [w402 w405] -> w9
    tunnel: w8 -> [w401 w404]
    tunnel: [w401 w403] -> w7
    frame False {
    }
    frame True {
      n267 = case shown="\"On\"" w404 {
        tunnel: [WPI_SolenoidValue."Forward" ("FiringPin") WPI_SolenoidValue."Reverse" ("FiringPin") WPI_SolenoidValue."Forward" ("FiringPin") WPI_SolenoidValue."Reverse" ("FiringPin")] -> w403
        frame "Off", Default {
        }
        frame "On" {
        }
        frame "Reverse" {
        }
        frame "Forward" {
        }
      }
      n268 = Tick Count (ms)() -> (millisecond timer value=w405:u32)
    }
  }
  n269 = case shown="True" w13 {
    tunnel: w3 -> [w411 _]
    tunnel: [w411 w414] -> w6
    tunnel: w4 -> [w410 w413]
    tunnel: [w410 w412] -> w5
    frame False {
    }
    frame True {
      n270 = case shown="\"On\"" w413 {
        tunnel: [WPI_SolenoidValue."Forward" ("FiringPin") WPI_SolenoidValue."Reverse" ("FiringPin") WPI_SolenoidValue."Forward" ("FiringPin") WPI_SolenoidValue."Reverse" ("FiringPin")] -> w412
        frame "Off", Default {
        }
        frame "On" {
        }
        frame "Reverse" {
        }
        frame "Forward" {
        }
      }
      n271 = Tick Count (ms)() -> (millisecond timer value=w414:u32)
    }
  }
  n272 = case shown="True" w42 {
    tunnel: w46 -> [_ w422]
    frame False {
      n273 = call <vilib>:"WPI_MotorControlRefNum Registry Get.vi"("refnum name"="Fisher Price") -> ("MotorControlDevRef"=w420:T12)  [unwired: 9 in, 1 out]
      n274 = call <vilib>:"WPI_MotorControlSetOutput.vi"("Output"=0.0, "MotorControlDevRef"=w420) -> ()  [unwired: 7 in, 3 out]
    }
    frame True {
      n275 = call <vilib>:"WPI_MotorControlRefNum Registry Get.vi"("refnum name"="Fisher Price") -> ("MotorControlDevRef"=w424:T12)  [unwired: 9 in, 1 out]
      n276 = call <vilib>:"WPI_MotorControlSetOutput.vi"("Output"=w422, "MotorControlDevRef"=w424) -> ()  [unwired: 7 in, 3 out]
    }
  }
  n277 = call <vilib>:"WPI_JoystickRefNum Registry Get.vi"("refnum name"="Joystick 1") -> ("JoystickDevRef"=w174:T10)  [unwired: 1 in, 9 out]
  n278 = call <vilib>:"WPI_JoystickGet.vi"("JoystickDevRef"=w174) -> ("Buttons"=w172:T22, "Axes"=w169:T38)  [unwired: 1 in, 4 out]
  n279 = Bundle By Name(cluster=w1, "PullBack"=w22, "FiringPin"=w7, "Grabber"=w5) -> (w24:T2)
  n280 = Bundle By Name(cluster=w28, "Button 1"=w26, "Button 2"=w9, "Button 3"=w6) -> (w25:T3)
  n281 = Unbundle By Name(w169) -> ("axis 1 (x)"=w150:dbl, "axis 2 (y)"=w148:dbl)  [unwired: 1 out]
  n282 = Cluster To Array(cluster=w169) -> (array=w168:dbl[])
  n283 = Cluster To Array(cluster=w172) -> (array=w171:bool[])
  n284 = local write "TimingForCopilot"(w25) -> ()
  n285 = local write "ManualOverridePistonStates"(w24) -> ()
  n286 = Negate(x=w150) -> (-x=w149:dbl)
  n287 = Negate(x=w148) -> (-x=w147:dbl)
  n288 = case shown="True" w77 {
    tunnel: w149 -> [_ w426]
    tunnel: w147 -> [_ w425]
    frame False {
    }
    frame True {
      n289 = call <vilib>:"WPI_RobotDriveRefNum Registry Get.vi"("refnum name"="Left and Right Motors") -> ("RobotDriveDevRef"=w429:T39)  [unwired: 1 in, 9 out]
      n290 = call <vilib>:"WPI_RobotDriveArcadeDrive_Standard(NoSaturation).vi"("Y axis value"=w425, "X axis value"=w426, "RobotDriveDevRef"=w429) -> ("Motor Values"=w427:dbl[])  [unwired: 1 in, 7 out]
      n291 = call <vilib>:"SD Write Numeric Array.vi"("Numeric Array"=w427, "Name"="Robot Drive Motors") -> ()  [unwired: 8 in, 2 out]
    }
  }
  n292 = call <vilib>:"SD Write Numeric Array.vi"("Numeric Array"=w168, "Name"="Joystick 1/Axes") -> ()  [unwired: 8 in, 2 out]
  n293 = call <vilib>:"SD Write Boolean Array.vi"("Boolean Array"=w171, "Name"="Joystick 1/Buttons") -> ()  [unwired: 8 in, 2 out]
